vi "Test Subscriber.vi"() -> ()   [LabVIEW 2021]
uses:
  ChannelCommon/typedef/FIFO Config.ctl
  ChannelCommon/ChannelCommon.lvlib
  CIFChannels/Typedef/Direction.ctl
  CIFChannels/CIFChannels.lvclass
  CIF_NIChn_Fifo_DAQ.lvclass
  D:/dev/Packages/Channel_Manager/src/CIFChannels/CIFChannels.lvclass
  ChannelCommon/typedef/Datatype Waveform.ctl
panel:
  in  "stop":bool
  out "timed out?":bool
  out "DAQ Out":T1[](array[typedef])
  out "error out":errorcluster
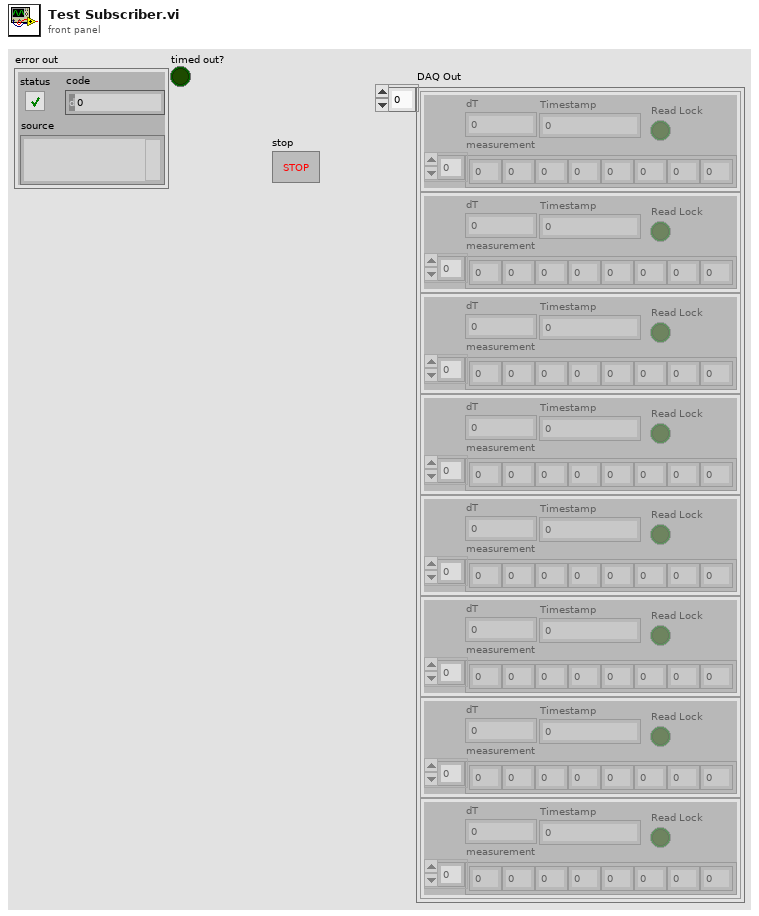
[diagram p1: front panel]
types:
  T1 = typedef "ChannelCommon.lvlib/Datatype Waveform.ctl" = cluster{"measurement":dbl[], "dT":dbl, "Timestamp":i64, "Read Lock":bool}
  T2 = typedef "ChannelCommon.lvlib/FIFO Config.ctl" = cluster{"Max Bytes/Msg":u64, "Max Msg/FIFO":u64, "Flags":u64}
  T3 = typedef "CIFChannels.lvclass/Direction.ctl" = enum16{"Publisher", "Subscriber"}
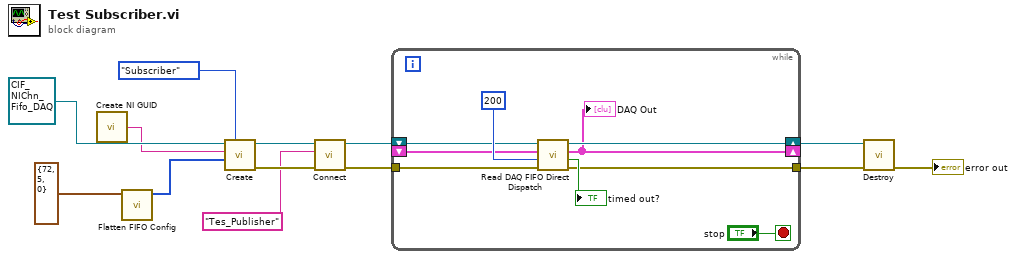
[diagram p0: block diagram]
diagram:
  n1 = call <vilib>:"Create NI GUID.vi"() -> ("NI GUID"=w7:string)
  n2 = call "Flatten FIFO Config.vi"("FIFO Config in"=T2 {"Max Bytes/Msg"=72, "Max Msg/FIFO"=5, "Flags"=0}) -> ("Flattened FIFO Config"=w1:u8[])  [unwired: 10 in]
  n3 = call-dynamic "Create.vi"("Direction"=Direction."Subscriber", "Custom Config Data"=w1, "Name"=w7, "CIFTag in"=refnum<class "CIF_NIChn_Fifo_DAQ.lvclass"> refnum ("CIF_NIChn_Fifo_Power.lvclass")) -> ("error out"=w10:errorcluster, "CIFTag out"=w11:refnum<class "CIF_NIChn_Fifo_DAQ.lvclass">)  [unwired: 6 in]
  n4 = call-dynamic "Connect.vi"("error in (no error)"=w10, "Connection Name"="Tes_Publisher", "CIFTag in"=w11) -> ("error out"=w3:errorcluster, "CIFTag out"=w6:refnum<class "CIF_NIChn_Fifo_DAQ.lvclass">)  [unwired: 7 in]
  n5 = while {
    shift-right: [w22] -> w13
    shift-left: w6 -> [w20]
    tunnel: w3 -> [w19]
    tunnel: [w17] -> w2
    shift-right: [w15] -> _
    shift-left: _ -> [w14]
    stop <- "stop" stop-if-true
    n6 = call "Read DAQ FIFO Direct Dispatch.vi"("error in (no error)"=w19, "Timeout (ms)"=200, "DAQ In"=w14, "CIFTag in"=w20) -> ("error out"=w17:errorcluster, "timed out?"=→"timed out?":bool, "DAQ Out"=w15:T1[], "CIFTag out"=w22:refnum<class "CIF_NIChn_Fifo_DAQ.lvclass">)  [unwired: 3 in, 1 out]
    "DAQ Out" <- w15
  }
  n7 = call-dynamic "Destroy.vi"("error in (no error)"=w2, "CIF_NIChn_Fifo_Power_DVR in"=w13) -> ("error out"=→"error out":errorcluster)  [unwired: 8 in, 1 out]
